vi "Polygon Intersection_Find Pockets.vi"(8 "y2":dbl[](array[numeric]), 9 "x2":dbl[](array[numeric]), 10 "y1":dbl[](array[numeric]), 11 "x1":dbl[](array[numeric])) -> (1 "index2":i32[](array[numeric]), 2 "index1":i32[](array[numeric]), 3 "left turn?":bool[](array[boolean]), 4 "inner?":bool, 5 "complex or concave?":bool)   [LabVIEW 2017, in "NI_AAL_Geometry.lvlib"]
uses:
  <vilib>/Analysis/NI_AAL_Geometry.lvlib
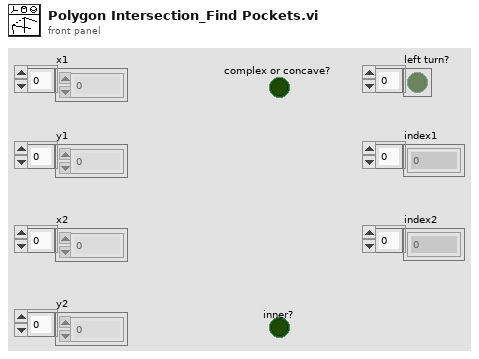
[diagram p1: front panel]
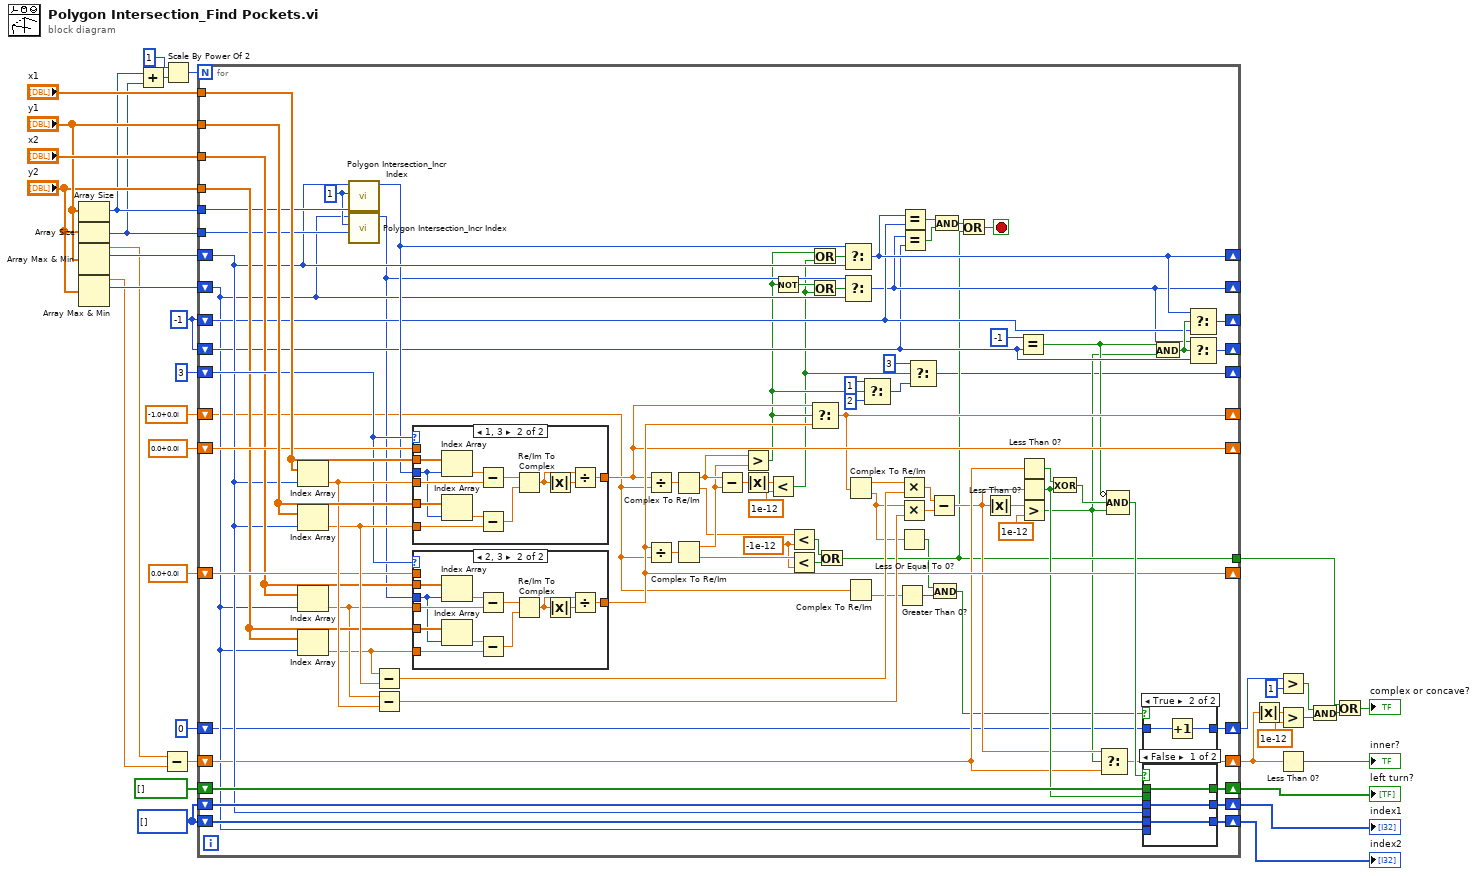
[diagram p0: block diagram]
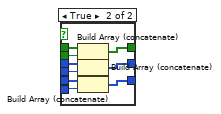
[diagram p5: hidden frame]
diagram:
  w17 = -1
  w36 = i32[] []
  n1 = Array Size(array="y1") -> (size(s)=w16:i32)
  n2 = Array Size(array="y2") -> (size(s)=w15:i32)
  n3 = Array Max & Min(array="y1") -> (max value=w22:dbl, max index (indices)=w34:i32)  [unwired: 2 out]
  n4 = Array Max & Min(array="y2") -> (max value=w23:dbl, max index (indices)=w33:i32)  [unwired: 2 out]
  n5 = Add(x=w16, y=w15) -> (x+y=w14:i32)
  n6 = Subtract(x=w22, y=w23) -> (x-y=w30:dbl)
  n7 = Scale By Power Of 2(n=1, x=w14) -> (x*2^n=w13:i32)
  n8 = for {
    N: w13 -> [_]
    shift-right: [w74] -> _
    shift-left: w34 -> [w85]
    shift-right: [w72] -> _
    shift-left: w33 -> [w56]
    tunnel: "x2" -> [w99]
    tunnel: "x1" -> [w110]
    tunnel: "y1" -> [w109]
    tunnel: "y2" -> [w98]
    shift-right: [w80] -> w2
    shift-left: w30 -> [w79]
    shift-right: [w120] -> w19
    shift-left: w36 -> [w122]
    shift-right: [w119] -> w18
    shift-left: w36 -> [w121]
    shift-right: [w115] -> w20
    shift-left: bool[] [] -> [w118]
    tunnel: w16 -> [w89]
    tunnel: w15 -> [w88]
    tunnel: [w64] -> w4
    shift-right: [w51] -> _
    shift-left: 3 -> [w100]
    shift-right: [w92] -> _
    shift-left: cdb 0.0+0.0i -> [w108]
    shift-right: [w93] -> _
    shift-left: cdb 0.0+0.0i -> [w101]
    shift-right: [w91] -> _
    shift-left: cdb -1.0+0.0i -> [w47]
    shift-right: [w77] -> _
    shift-left: w17 -> [w73]
    shift-right: [w76] -> _
    shift-left: w17 -> [w69]
    shift-right: [w40] -> w10
    shift-left: 0 -> [w42]
    stop <- w66 stop-if-true
    w37 = -1e-12
    w83 = 1 ("incr")
    n9 = Index Array(array=w110, index=w85) -> (element=w103:dbl)
    n10 = Index Array(array=w109, index=w85) -> (element=w102:dbl)
    n11 = Index Array(array=w99, index=w56) -> (element=w97:dbl)
    n12 = Index Array(array=w98, index=w56) -> (element=w96:dbl)
    n13 = call <vilib>:"Polygon Intersection_Incr Index.vi"("polygon size"=w89, "incr"=w83, "index"=w85) -> ("incr index"=w84:i32)  [unwired: 8 in]
    n14 = call <vilib>:"Polygon Intersection_Incr Index.vi"("polygon size"=w88, "incr"=w83, "index"=w56) -> ("incr index"=w55:i32)  [unwired: 8 in]
    n15 = Subtract(x=w96, y=w102) -> (x-y=w116:dbl)
    n16 = Subtract(x=w97, y=w103) -> (x-y=w117:dbl)
    n17 = case shown="1, 3" w100 {
      tunnel: w110 -> [_ w150]
      tunnel: w109 -> [_ w151]
      tunnel: [w139 w145] -> w92
      tunnel: w108 -> [w139 _]
      tunnel: w103 -> [_ w143]
      tunnel: w102 -> [_ w141]
      tunnel: w84 -> [_ w140]
      frame 0, Default {
      }
      frame 1, 3 {
        n18 = Index Array(array=w150, index=w140) -> (element=w144:dbl)
        n19 = Index Array(array=w151, index=w140) -> (element=w142:dbl)
        n20 = Subtract(x=w144, y=w143) -> (x-y=w149:dbl)
        n21 = Subtract(x=w142, y=w141) -> (x-y=w148:dbl)
        n22 = Re/Im To Complex(1:w148, 2:w149) -> (0:w147:cdb)
        n23 = Absolute Value(x=w147) -> (abs(x)=w146:dbl)
        n24 = Divide(x=w147, y=w146) -> (x/y=w145:cdb)
      }
    }
    n25 = case shown="2, 3" w100 {
      tunnel: w99 -> [_ w137]
      tunnel: w98 -> [_ w138]
      tunnel: [w126 w132] -> w93
      tunnel: w101 -> [w126 _]
      tunnel: w97 -> [_ w130]
      tunnel: w96 -> [_ w128]
      tunnel: w55 -> [_ w127]
      frame 0, Default {
      }
      frame 2, 3 {
        n26 = Index Array(array=w137, index=w127) -> (element=w131:dbl)
        n27 = Index Array(array=w138, index=w127) -> (element=w129:dbl)
        n28 = Subtract(x=w131, y=w130) -> (x-y=w136:dbl)
        n29 = Subtract(x=w129, y=w128) -> (x-y=w135:dbl)
        n30 = Re/Im To Complex(1:w135, 2:w136) -> (0:w134:cdb)
        n31 = Absolute Value(x=w134) -> (abs(x)=w133:dbl)
        n32 = Divide(x=w134, y=w133) -> (x/y=w132:cdb)
      }
    }
    n33 = Divide(x=w92, y=w47) -> (x/y=w107:cdb)
    n34 = Divide(x=w93, y=w47) -> (x/y=w106:cdb)
    n35 = Complex To Re/Im(x + iy=w107) -> (x=w61:dbl, y=w38:dbl)
    n36 = Complex To Re/Im(x + iy=w106) -> (x=w60:dbl, y=w39:dbl)
    n37 = Subtract(x=w61, y=w60) -> (x-y=w59:dbl)
    n38 = Greater?(x=w61, y=w60) -> (0:w52:bool)
    n39 = Absolute Value(x=w59) -> (abs(x)=w58:dbl)
    n40 = Less?(x=w58, y=1e-12) -> (x < y?=w49:bool)
    n41 = Not(x=w52) -> (.not. x?=w53:bool)
    n42 = Less?(x=w38, y=w37) -> (x < y?=w105:bool)
    n43 = Less?(x=w39, y=w37) -> (x < y?=w104:bool)
    n44 = Or(x=w52, y=w49) -> (x .or. y?=w62:bool)
    n45 = Or(x=w53, y=w49) -> (x .or. y?=w54:bool)
    n46 = Select(t=w92, s=w52, f=w93) -> (s? t:f=w91:cdb)
    n47 = Or(x=w105, y=w104) -> (x .or. y?=w64:bool)
    n48 = Select(t=w84, s=w62, f=w85) -> (s? t:f=w74:i32)
    n49 = Select(t=w55, s=w54, f=w56) -> (s? t:f=w72:i32)
    n50 = Complex To Re/Im(x + iy=w91) -> (x=w90:dbl, y=w45:dbl)
    n51 = Complex To Re/Im(x + iy=w47) -> (y=w46:dbl)  [unwired: 1 out]
    n52 = Select(t=1, s=w52, f=2) -> (s? t:f=w50:i32)
    n53 = Greater Than 0?(x=w46) -> (x > 0?=w43:bool)
    n54 = Multiply(x=w90, y=w116) -> (x*y=w94:dbl)
    n55 = Multiply(x=w45, y=w117) -> (x*y=w95:dbl)
    n56 = Less Or Equal To 0?(x=w45) -> (x <= 0?=w44:bool)
    n57 = Equal?(x=w74, y=w73) -> (x = y?=w71:bool)
    n58 = Equal?(x=w72, y=w69) -> (x = y?=w70:bool)
    n59 = Select(t=3 ("f"), s=w49, f=w50) -> (s? t:f=w51:i32)
    n60 = Subtract(x=w94, y=w95) -> (x-y=w78:dbl)
    n61 = And(x=w44, y=w43) -> (x .and. y?=w41:bool)
    n62 = And(x=w71, y=w70) -> (x .and. y?=w65:bool)
    n63 = Or(x=w65, y=w64) -> (x .or. y?=w66:bool)
    n64 = Absolute Value(x=w78) -> (abs(x)=w114:dbl)
    n65 = Equal?(x=-1 ("y"), y=w69) -> (x = y?=w67:bool)
    n66 = Less Than 0?(x=w79) -> (x < 0?=w82:bool)
    n67 = Less Than 0?(x=w78) -> (x < 0?=w81:bool)
    n68 = Greater?(x=w114, y=1e-12) -> (0:w63:bool)
    n69 = Exclusive Or(1:w81, 2:w82) -> (0:w112:bool)
    n70 = Select(t=w78, s=w63, f=w79) -> (s? t:f=w80:dbl)
    n71 = Compound Arithmetic op=AND(invert w67, w112, w63) -> (w111:bool)
    n72 = case shown="True" w41 {
      tunnel: w42 -> [w123 w125]
      tunnel: [w123 w124] -> w40
      frame False {
      }
      frame True {
        n73 = Increment(x=w125) -> (x+1=w124:i32)
      }
    }
    n74 = case shown="False" w111 {
      tunnel: w56 -> [_ w155]
      tunnel: w122 -> [w154 w158]
      tunnel: w121 -> [w153 w156]
      tunnel: [w154 w163] -> w120
      tunnel: [w153 w162] -> w119
      tunnel: w118 -> [w152 w160]
      tunnel: [w152 w161] -> w115
      tunnel: w85 -> [_ w157]
      tunnel: w81 -> [_ w159]
      frame False {
      }
      frame True {
        n75 = Build Array (concatenate)(w160, w159) -> (w161:bool[])
        n76 = Build Array (concatenate)(w158, w157) -> (w163:i32[])
        n77 = Build Array (concatenate)(w156, w155) -> (w162:i32[])
      }
    }
    n78 = And(x=w67, y=w63) -> (x .and. y?=w75:bool)
    n79 = Select(t=w74, s=w75, f=w73) -> (s? t:f=w77:i32)
    n80 = Select(t=w72, s=w75, f=w69) -> (s? t:f=w76:i32)
  }
  "left turn?" <- w20
  "index1" <- w19
  "index2" <- w18
  n81 = Absolute Value(x=w2) -> (abs(x)=w1:dbl)
  n82 = Greater?(x=w10, y=1) -> (0:w6:bool)
  n83 = Greater?(x=w1, y=1e-12) -> (0:w7:bool)
  n84 = Less Than 0?(x=w2) -> (x < 0?=→"inner?":bool)
  n85 = And(x=w6, y=w7) -> (x .and. y?=w5:bool)
  n86 = Or(x=w4, y=w5) -> (x .or. y?=→"complex or concave?":bool)
